vi "1_3.vi"() -> ()   [LabVIEW 2018]
panel:
  in  "Delay Time (s)":dbl=0.25
  in  "stop":bool
  out "Table":string[][](table)
  out "Waveform Graph":dynamicdata(graph)
  out "Mean":dbl
  in  "Enable":bool=TRUE
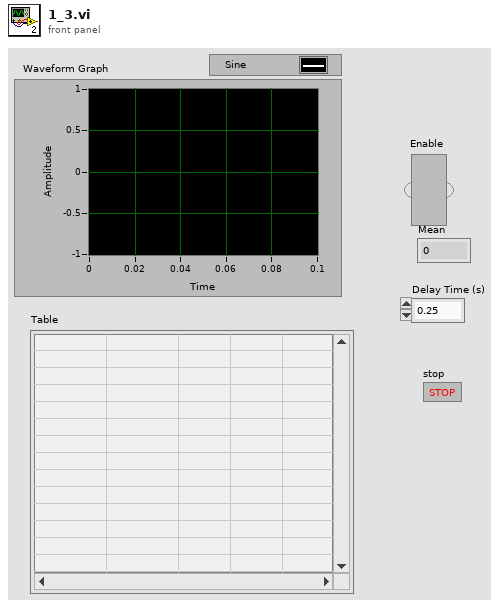
[diagram p1: front panel]
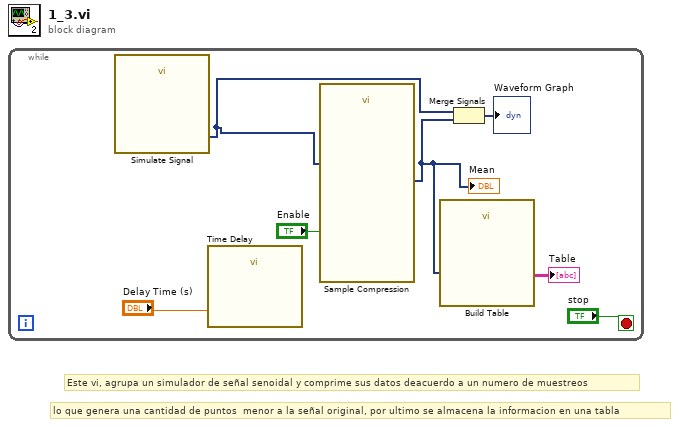
[diagram p0: block diagram]
diagram:
  # "lo que genera una cantidad de puntos  menor a la señal original, por ultimo se almacena la informacion en una tabla"
  # "Este vi, agrupa un simulador de señal senoidal y comprime sus datos deacuerdo a un numero de muestreos"
  n1 = while {
    stop <- "stop" stop-if-true
    n2 = call "Simulate Signal"() -> ("Sine"=w2:dynamicdata)  [unwired: 14 in, 1 out]
    n3 = call "Time Delay"("Delay Time (s)"="Delay Time (s)") -> ()  [unwired: 10 in, 1 out]
    n4 = call "Sample Compression"("Enable"="Enable", "Signals"=w2) -> ("Mean"=w1:dynamicdata)  [unwired: 6 in, 3 out]
    "Mean" <- w1
    n5 = call "Build Table"("Signals"=w1) -> ("Table"=→"Table":string[][])  [unwired: 4 in, 6 out]
    n6 = Merge Signals(w2, w1) -> (→"Waveform Graph":dynamicdata)
  }
